vi "EVT Camera Get Int32Param Min.vi"(9 "min":i32, 10 "name":string, 11 "camera":u64) -> (1 "min out":i32, 3 "function return":u32(ring))   [LabVIEW 2019, in "EmergentCameraC.lvlib"]
doc: "EMERGENTCAMERAC_API EVT_ERROR EVT_CameraGetInt32ParamMin(Camera_Handle camera, const char* name, int* min);"
uses:
  EmergentCameraC.lvlib
  emergentInstall_Windows/win64/eSDK/bin/EmergentCameraC.dll
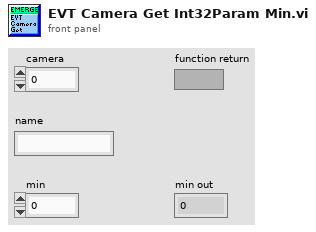
[diagram p1: front panel]
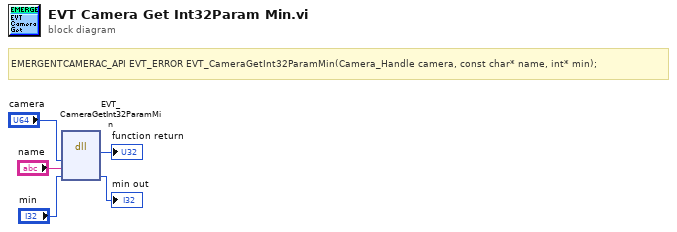
[diagram p0: block diagram]
diagram:
  # "EMERGENTCAMERAC_API EVT_ERROR EVT_CameraGetInt32ParamMin(Camera_Handle camera, const char* name, int* min);"
  n1 = dll-call lib="E:/emergent/host-new_QT/emergentInstall_Windows/win64/eSDK/bin/EmergentCameraC.*" fn="EVT_CameraGetInt32ParamMin"("camera"="camera", "name"="name", "min"="min") -> (→"function return":u32, "min"=→"min out":i32)  [unwired: 5 in, 2 out]
